vi "SetResponder.vi"(8 "error in (no error)":errorcluster, 9 "Responder":refnum<class "BaseResponder.lvclass">, 11 "MultiResponder in":refnum<class "MultiResponder.lvclass">) -> (0 "error out":errorcluster, 3 "MultiResponder out":refnum<class "MultiResponder.lvclass">)   [LabVIEW 2013, in "MultiResponder.lvclass"]
doc: "Add a named child responder to the multi responder"
uses:
  MultiResponder.lvclass
  BaseResponder/BaseResponder.lvclass
  MultiResponder.lvclass/MultiResponder.ctl
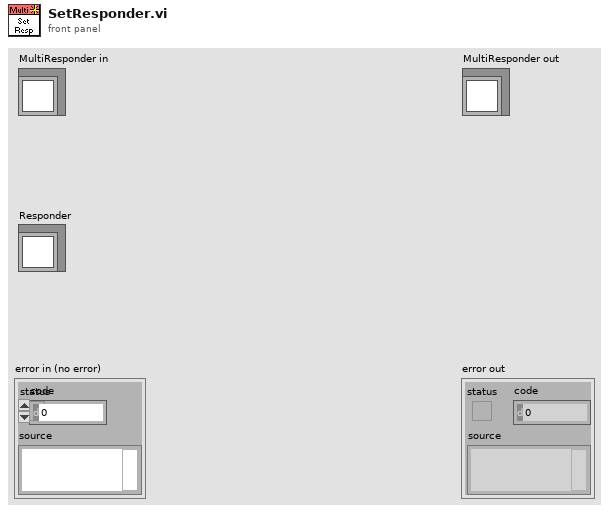
[diagram p1: front panel]
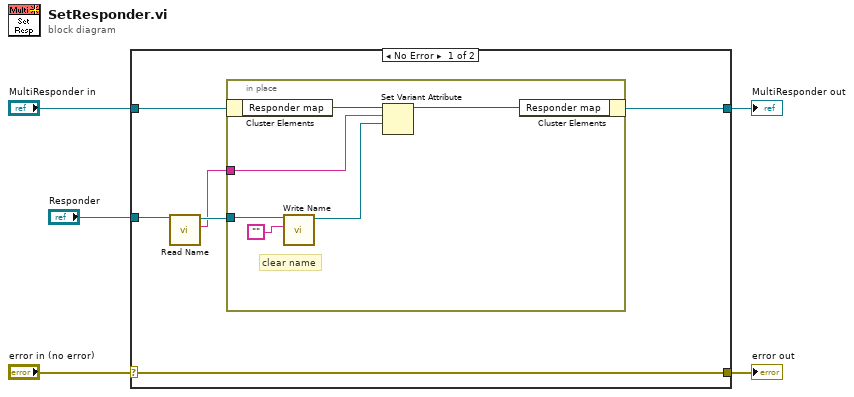
[diagram p0: block diagram]
diagram:
  n1 = case shown="No Error" "error in (no error)" {
    selector: "error in (no error)" -> [w11 w19]
    tunnel: [w11 w19] -> w4
    tunnel: [w6 w18] -> w2
    tunnel: "MultiResponder in" -> [w10 w18]
    tunnel: "Responder" -> [w9 _]
    frame No Error {
      n2 = call "Read Name.vi"("BaseResponder in"=w9) -> ("Name"=w7:string, "BaseResponder out"=w8:refnum<class "BaseResponder.lvclass">)  [unwired: 8 in, 1 out]
      n3 = in-place "In Place Element Structure" {
        in-place-border: w7 -> [w16]
        in-place-border: w8 -> [w15]
        # "clear name"
        n4 = in-place-cluster #1(w10) -> ("Responder map"=w17:variant)
        n5 = call "Write Name.vi"("Name"="", "BaseResponder in"=w15) -> ("BaseResponder out"=w13:refnum<class "BaseResponder.lvclass">)  [unwired: 8 in, 1 out]
        n6 = Set Variant Attribute(Variant=w17, name=w16, value=w13) -> (Variant out=w12:variant)  [unwired: 1 in, 2 out]
        n7 = in-place-cluster #1("Responder map"=w12) -> (w6:refnum<class "MultiResponder.lvclass">)
      }
    }
    frame Error {
    }
  }
  "error out" <- w4
  "MultiResponder out" <- w2
